vi "Write previous pwl scale.vi"(8 "error in (no error)":errorcluster caption="에러 입력(에러 없음)", 10 "previous pwl scale":dbl=1.0, 11 "PWL 입력":refnum<class "PWL.lvclass">) -> (0 "error out":errorcluster caption="에러 출력", 3 "PWL 출력":refnum<class "PWL.lvclass">)   [LabVIEW 2020, in "PWL.lvclass"]
uses:
  PWL.lvclass
  PWL.lvclass/PWL.ctl
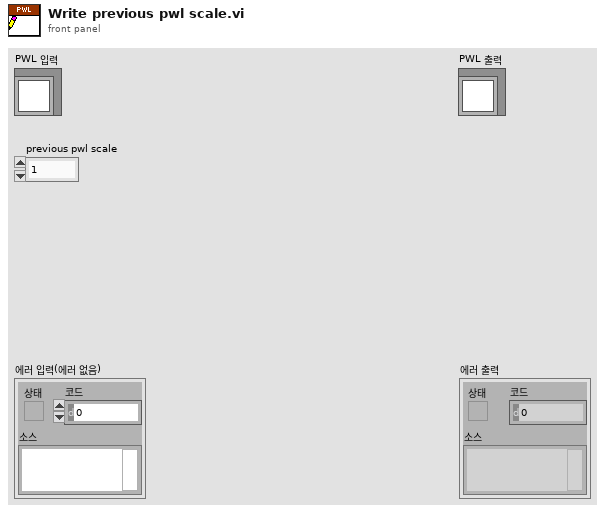
[diagram p1: front panel]
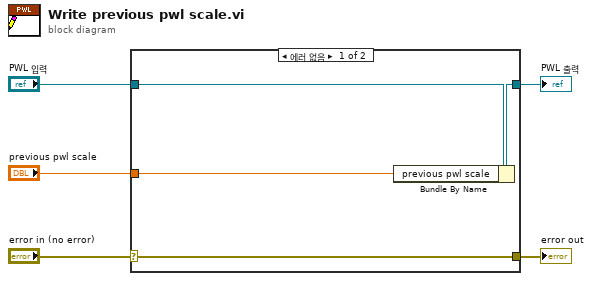
[diagram p0: block diagram]
diagram:
  n1 = case shown="에러 없음" "error in (no error)" {
    selector: "error in (no error)" -> [w9 w10]
    tunnel: [w9 w10] -> w4
    tunnel: [w7 w11] -> w2
    tunnel: "PWL 입력" -> [w8 w11]
    tunnel: "previous pwl scale" -> [w6 _]
    frame No Error {
      n2 = Bundle By Name(cluster=w8, "previous pwl scale"=w6) -> (w7:refnum<class "PWL.lvclass">)
    }
    frame Error {
    }
  }
  "error out" <- w4
  "PWL 출력" <- w2
